vi "簇转换为数组.vi"() -> ()   [LabVIEW 2018]
panel:
  in  "停止":bool
  out "字符串数组":string[](array[string])
  out "数值数组":dbl[](array[numeric])
  in  "字符串簇":T1
  in  "数值簇":T2
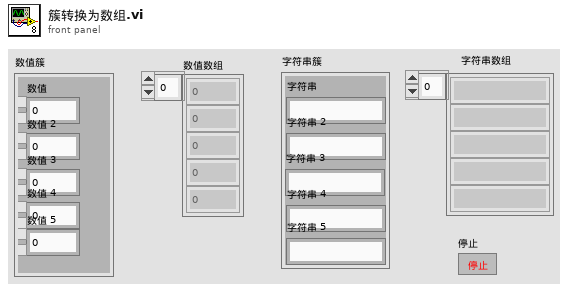
[diagram p1: front panel]
types:
  T1 = cluster{"字符串":string, "字符串 2":string, "字符串 3":string, "字符串 4":string, "字符串 5":string}
  T2 = cluster{"数值":dbl, "数值 2":dbl, "数值 3":dbl, "数值 4":dbl, "数值 5":dbl}
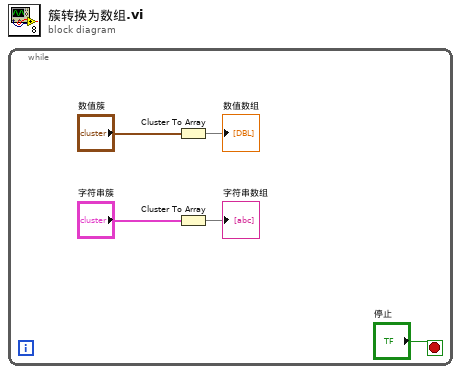
[diagram p0: block diagram]
diagram:
  n1 = while {
    stop <- "停止" stop-if-true
    n2 = Cluster To Array(cluster="数值簇") -> (array=→"数值数组":dbl[])
    n3 = Cluster To Array(cluster="字符串簇") -> (array=→"字符串数组":string[])
  }
